vi "Complex Dot Product PtByPt.vi"(2 "initialize":bool, 3 "sample length":i32=100, 4 "x":cdb format="%#.6g", 5 "y":cdb format="%#.6g") -> (0 "error":i32, 1 "X*Y":cdb format="%#.6g")   [LabVIEW 2017, in "NI_PtbyPt.lvlib"]
doc: "Computes the dot product,<B> X*Y</B>, of the complex values <B>y</B> and <B>x</B>."
uses:
  <vilib>/ptbypt/NI_PtbyPt.lvlib
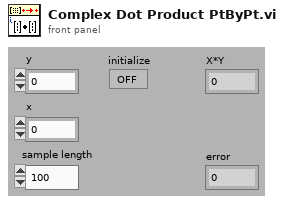
[diagram p1: front panel]
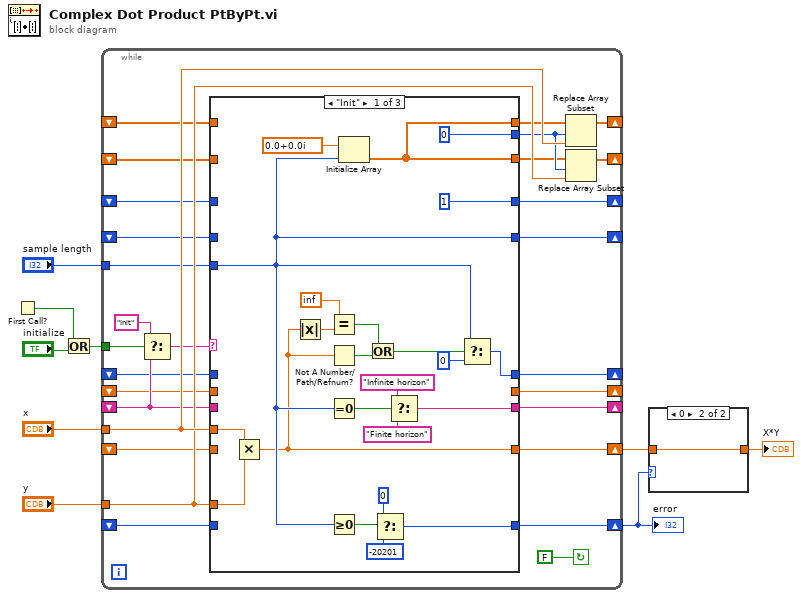
[diagram p0: block diagram]
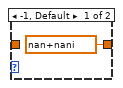
[diagram p2: hidden frame]
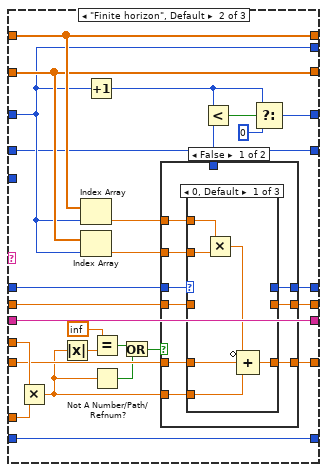
[diagram p3: hidden frame]
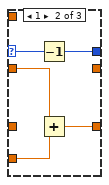
[diagram p4: hidden frame]
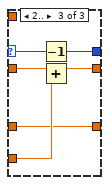
[diagram p5: hidden frame]
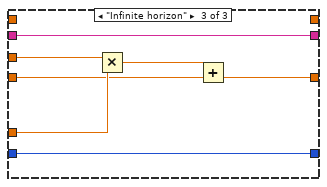
[diagram p7: hidden frame]
diagram:
  n1 = First Call?() -> (First Call?: T/F=w6:bool)
  n2 = Or(x=w6, y="initialize") -> (x .or. y?=w7:bool)
  n3 = while {
    tunnel: w7 -> [w23]
    shift-left: _ -> [w21]
    shift-right: [w19] -> _
    shift-left: _ -> [w24]
    shift-right: [w25] -> _
    shift-left: _ -> [w26]
    shift-right: [w27] -> w2
    shift-left: _ -> [w29]
    shift-right: [w15] -> _
    shift-left: _ -> [w28]
    shift-right: [w36] -> _
    shift-left: _ -> [w32]
    shift-right: [w37] -> _
    tunnel: "x" -> [w35]
    tunnel: "y" -> [w34]
    tunnel: "sample length" -> [w17]
    shift-right: [w16] -> w3
    shift-left: _ -> [w10]
    shift-right: [w14] -> _
    shift-left: _ -> [w13]
    shift-right: [w12] -> _
    shift-left: _ -> [w11]
    stop <- FALSE continue-if-true
    n4 = Select(t="Init", s=w23, f=w21) -> (s? t:f=w20:string)
    n5 = case shown="\"Init\"" w20 {
      tunnel: w34 -> [w59 w65 w120]
      tunnel: w35 -> [w60 w86 w121]
      tunnel: [1 w80 _] -> w15
      tunnel: [0 ("Index") w77 _] -> w33
      tunnel: w24 -> [_ w69 _]
      tunnel: w32 -> [_ w81 _]
      tunnel: [w55 w81 _] -> w31
      tunnel: [w55 w79 _] -> w30
      tunnel: w29 -> [_ w77 _]
      tunnel: w28 -> [_ w79 _]
      tunnel: [w43 w76 w119] -> w27
      tunnel: w26 -> [_ w75 w117]
      tunnel: [w46 w69 _] -> w25
      tunnel: [w51 w74 w118] -> w19
      tunnel: w21 -> [_ w74 w118]
      tunnel: w17 -> [w46 _ _]
      tunnel: [w47 w68 w115] -> w16
      tunnel: [w45 w73 _] -> w14
      tunnel: w13 -> [_ w72 _]
      tunnel: [_ w71 _] -> w12
      tunnel: w11 -> [_ w70 _]
      tunnel: w10 -> [_ w68 w115]
      frame "Init" {
        n6 = Multiply(x=w60, y=w59) -> (x*y=w43:cdb)
        n7 = Absolute Value(x=w43) -> (abs(x)=w42:dbl)
        n8 = Equal?(x=inf, y=w42) -> (x = y?=w40:bool)
        n9 = Not A Number/Path/Refnum?(number/path/refnum=w43) -> (NaN/Path/Refnum?=w39:bool)
        n10 = Equal To 0?(x=w46) -> (x = 0?=w54:bool)
        n11 = Greater Or Equal To 0?(x=w46) -> (x >= 0?=w50:bool)
        n12 = Initialize Array(cdb 0.0+0.0i ("Element Data"), w46) -> (w55:cdb[])
        n13 = Or(x=w40, y=w39) -> (x .or. y?=w38:bool)
        n14 = Select(t=0, s=w50, f=-20201) -> (s? t:f=w47:i32)
        n15 = Select(t="Infinite horizon", s=w54, f="Finite horizon") -> (s? t:f=w51:string)
        n16 = Select(t=w46, s=w38, f=0) -> (s? t:f=w45:i32)
      }
      frame "Finite horizon", Default {
        n17 = Multiply(x=w86, y=w65) -> (x*y=w64:cdb)
        n18 = Absolute Value(x=w64) -> (abs(x)=w67:dbl)
        n19 = Index Array(array=w81, index=w77) -> (element=w82:cdb)
        n20 = Index Array(array=w79, index=w77) -> (element=w78:cdb)
        n21 = Increment(x=w77) -> (x+1=w84:i32)
        n22 = Equal?(x=inf, y=w67) -> (x = y?=w63:bool)
        n23 = Not A Number/Path/Refnum?(number/path/refnum=w64) -> (NaN/Path/Refnum?=w62:bool)
        n24 = Or(x=w63, y=w62) -> (x .or. y?=w61:bool)
        n25 = case shown="False" w61 {
          tunnel: w82 -> [w95 _]
          tunnel: w78 -> [w94 _]
          tunnel: [w93 w114] -> w76
          tunnel: w75 -> [w92 _]
          tunnel: w64 -> [w91 w114]
          tunnel: [w90 w113] -> w73
          tunnel: w72 -> [w89 _]
          tunnel: [w88 _] -> w71
          tunnel: w70 -> [w87 _]
          tunnel: w69 -> [_ w113]
          frame False {
            n26 = case shown="0, Default" w89 {
              selector: w89 -> [_ w106 w112]
              tunnel: w95 -> [w101 _ _]
              tunnel: w94 -> [w100 _ _]
              tunnel: [w99 w102 w107] -> w93
              tunnel: w92 -> [w98 _ w107]
              tunnel: w91 -> [w97 w104 w110]
              tunnel: [_ w105 w111] -> w90
              tunnel: [_ _ w109] -> w88
              tunnel: w87 -> [_ w103 w108]
              frame 0, Default {
                n27 = Multiply(x=w101, y=w100) -> (x*y=w96:cdb)
                n28 = Compound Arithmetic op=ADD(invert w96, w98, w97) -> (w99:cdb)
              }
              frame 1 {
                n29 = Decrement(x=w106) -> (x-1=w105:i32)
                n30 = Add(x=w103, y=w104) -> (x+y=w102:cdb)
              }
              frame 2.. {
                n31 = Decrement(x=w112) -> (x-1=w111:i32)
                n32 = Add(x=w108, y=w110) -> (x+y=w109:cdb)
              }
            }
          }
          frame True {
          }
        }
        n33 = Less?(x=w84, y=w69) -> (x < y?=w83:bool)
        n34 = Select(t=w84, s=w83, f=0 ("Index")) -> (s? t:f=w80:i32)
      }
      frame "Infinite horizon" {
        n35 = Multiply(x=w121, y=w120) -> (x*y=w116:cdb)
        n36 = Add(x=w116, y=w117) -> (x+y=w119:cdb)
      }
    }
    n37 = Replace Array Subset(array=w31, new element=w35, index=w33) -> (w37:cdb[])
    n38 = Replace Array Subset(array=w30, new element=w34, index=w33) -> (w36:cdb[])
  }
  "error" <- w3
  n39 = case shown="0" w3 {
    tunnel: w2 -> [_ w123]
    tunnel: [cdb nan+nani w123] -> w1
    frame -1, Default {
    }
    frame 0 {
    }
  }
  "X*Y" <- w1
